vi "Begin.vi"() -> (0 "error out":errorcluster)   [LabVIEW 2013]
doc: "Called before other user functions, this VI is expected to open initial I/O refnums, load in file data, and do all program initialization. Notice that the <B>error out</B> terminal is simply used for data flow. Wiring it to other structures or subVIs ensures that this VI runs first."
uses:
  <vilib>/Rock Robotics/WPI/DriverStation/WPI_DriverStationRobotMode2.ctl
  Specials/Global Data.vi
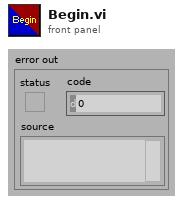
[diagram p1: front panel]
types:
  T1 = typedef "WPI_DriverStationRobotMode2.ctl" = enum16{"Autonomous Disabled", "Autonomous Enabled", "Teleop Disabled", "Teleop Enabled", "Timeout", "Finish", "Test Disabled", "Test Enabled"}
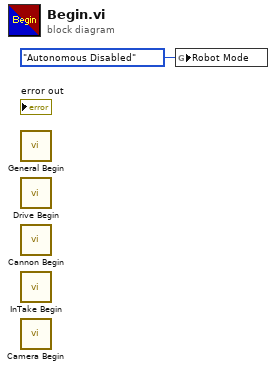
[diagram p0: block diagram]
diagram:
  n1 = call "General Begin.vi"() -> ()  [unwired: 12 in]
  n2 = call "Drive Begin.vi"() -> ()  [unwired: 12 in]
  n3 = call "Cannon Begin.vi"() -> ()  [unwired: 12 in]
  n4 = call "InTake Begin.vi"() -> ()  [unwired: 12 in]
  n5 = call "Camera Begin.vi"() -> ()  [unwired: 12 in]
  n6 = global write "Global Data.vi" "Robot Mode"(WPI_DriverStationRobotMode2."Autonomous Disabled" ("Robot Mode")) -> ()
